vi "DraggingDresser.vi"() -> ()   [LabVIEW 2014]
panel:
  out "Force":dbl[](array[numeric])
  out "Angle for Minimum Force":i32 format="%.1f"
  in  "Coefficient of Kinetic Friction":dbl format="%.1f"
  out "Waveform Graph":dbl[](graph)
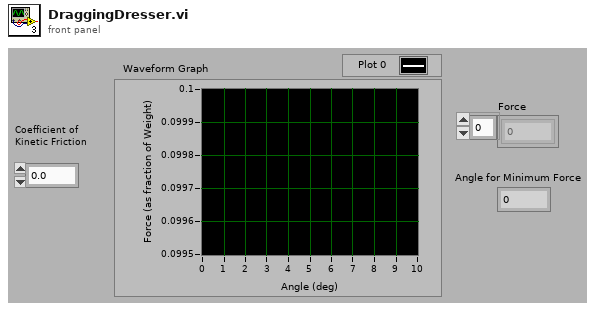
[diagram p1: front panel]
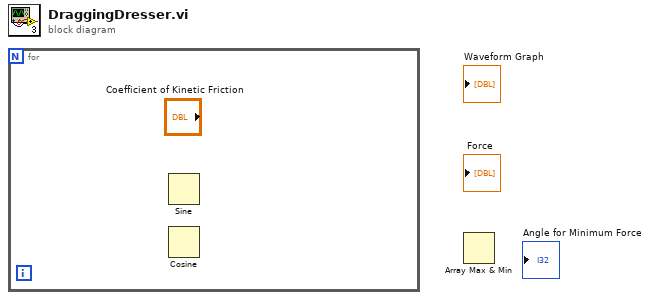
[diagram p0: block diagram]
diagram:
  n1 = for {
    n2 = Sine() -> ()  [unwired: 1 in, 1 out]
    n3 = Cosine() -> ()  [unwired: 1 in, 1 out]
  }
  n4 = Array Max & Min() -> ()  [unwired: 1 in, 4 out]
